vi "Flowmeter.vi"() -> ()   [LabVIEW 2017]
uses:
  Type Def/Data.ctl
  <vilib>/DAQmx/read.llb/DAQmx Read (Analog 2D DBL NChan NSamp).vi
  <vilib>/DAQmx/configure/timing.llb/DAQmx Timing (Sample Clock).vi
  <vilib>/DAQmx/miscellaneous.llb/DAQmx Fill In Error Info.vi
panel:
  out "valeur de l'horloge en ms":u32
  in  "Bouton Accueil":bool
  out "task out":refnum<k21>
  out "Type .EXE":bool
  out "sortie d'erreur 2":errorcluster caption="sortie d'erreur"
  out "error out":errorcluster
  out "Chaîne":string
  out "error IO":errorcluster
  out "sortie d'erreur":errorcluster
  in  "Start acquisition":bool
  out "High Voltage":dbl format="%#_2g"
  out "FLOW_SMC3":dbl caption="FLOW_AMP" format="%#.2g"
  out "FLOW_SMC2":dbl caption="FLOW_OSC" format="%#.2g"
  out "FLOW_SMC1":dbl caption="FLOW_BENCH" format="%#.2g"
  out "TEMP_SMC3":dbl caption="TEMP_AMP" format="%#.2g"
  out "TEMP_SMC2":dbl caption="TEMP_OSC" format="%#.2g"
  out "TEMP_SMC1":dbl caption="TEMP_BENCH" format="%#.2g"
  out "Flow data file (1sec)":refnum<file>
  out "Tableau":dbl[](array[numeric])
  in  "Stop":bool
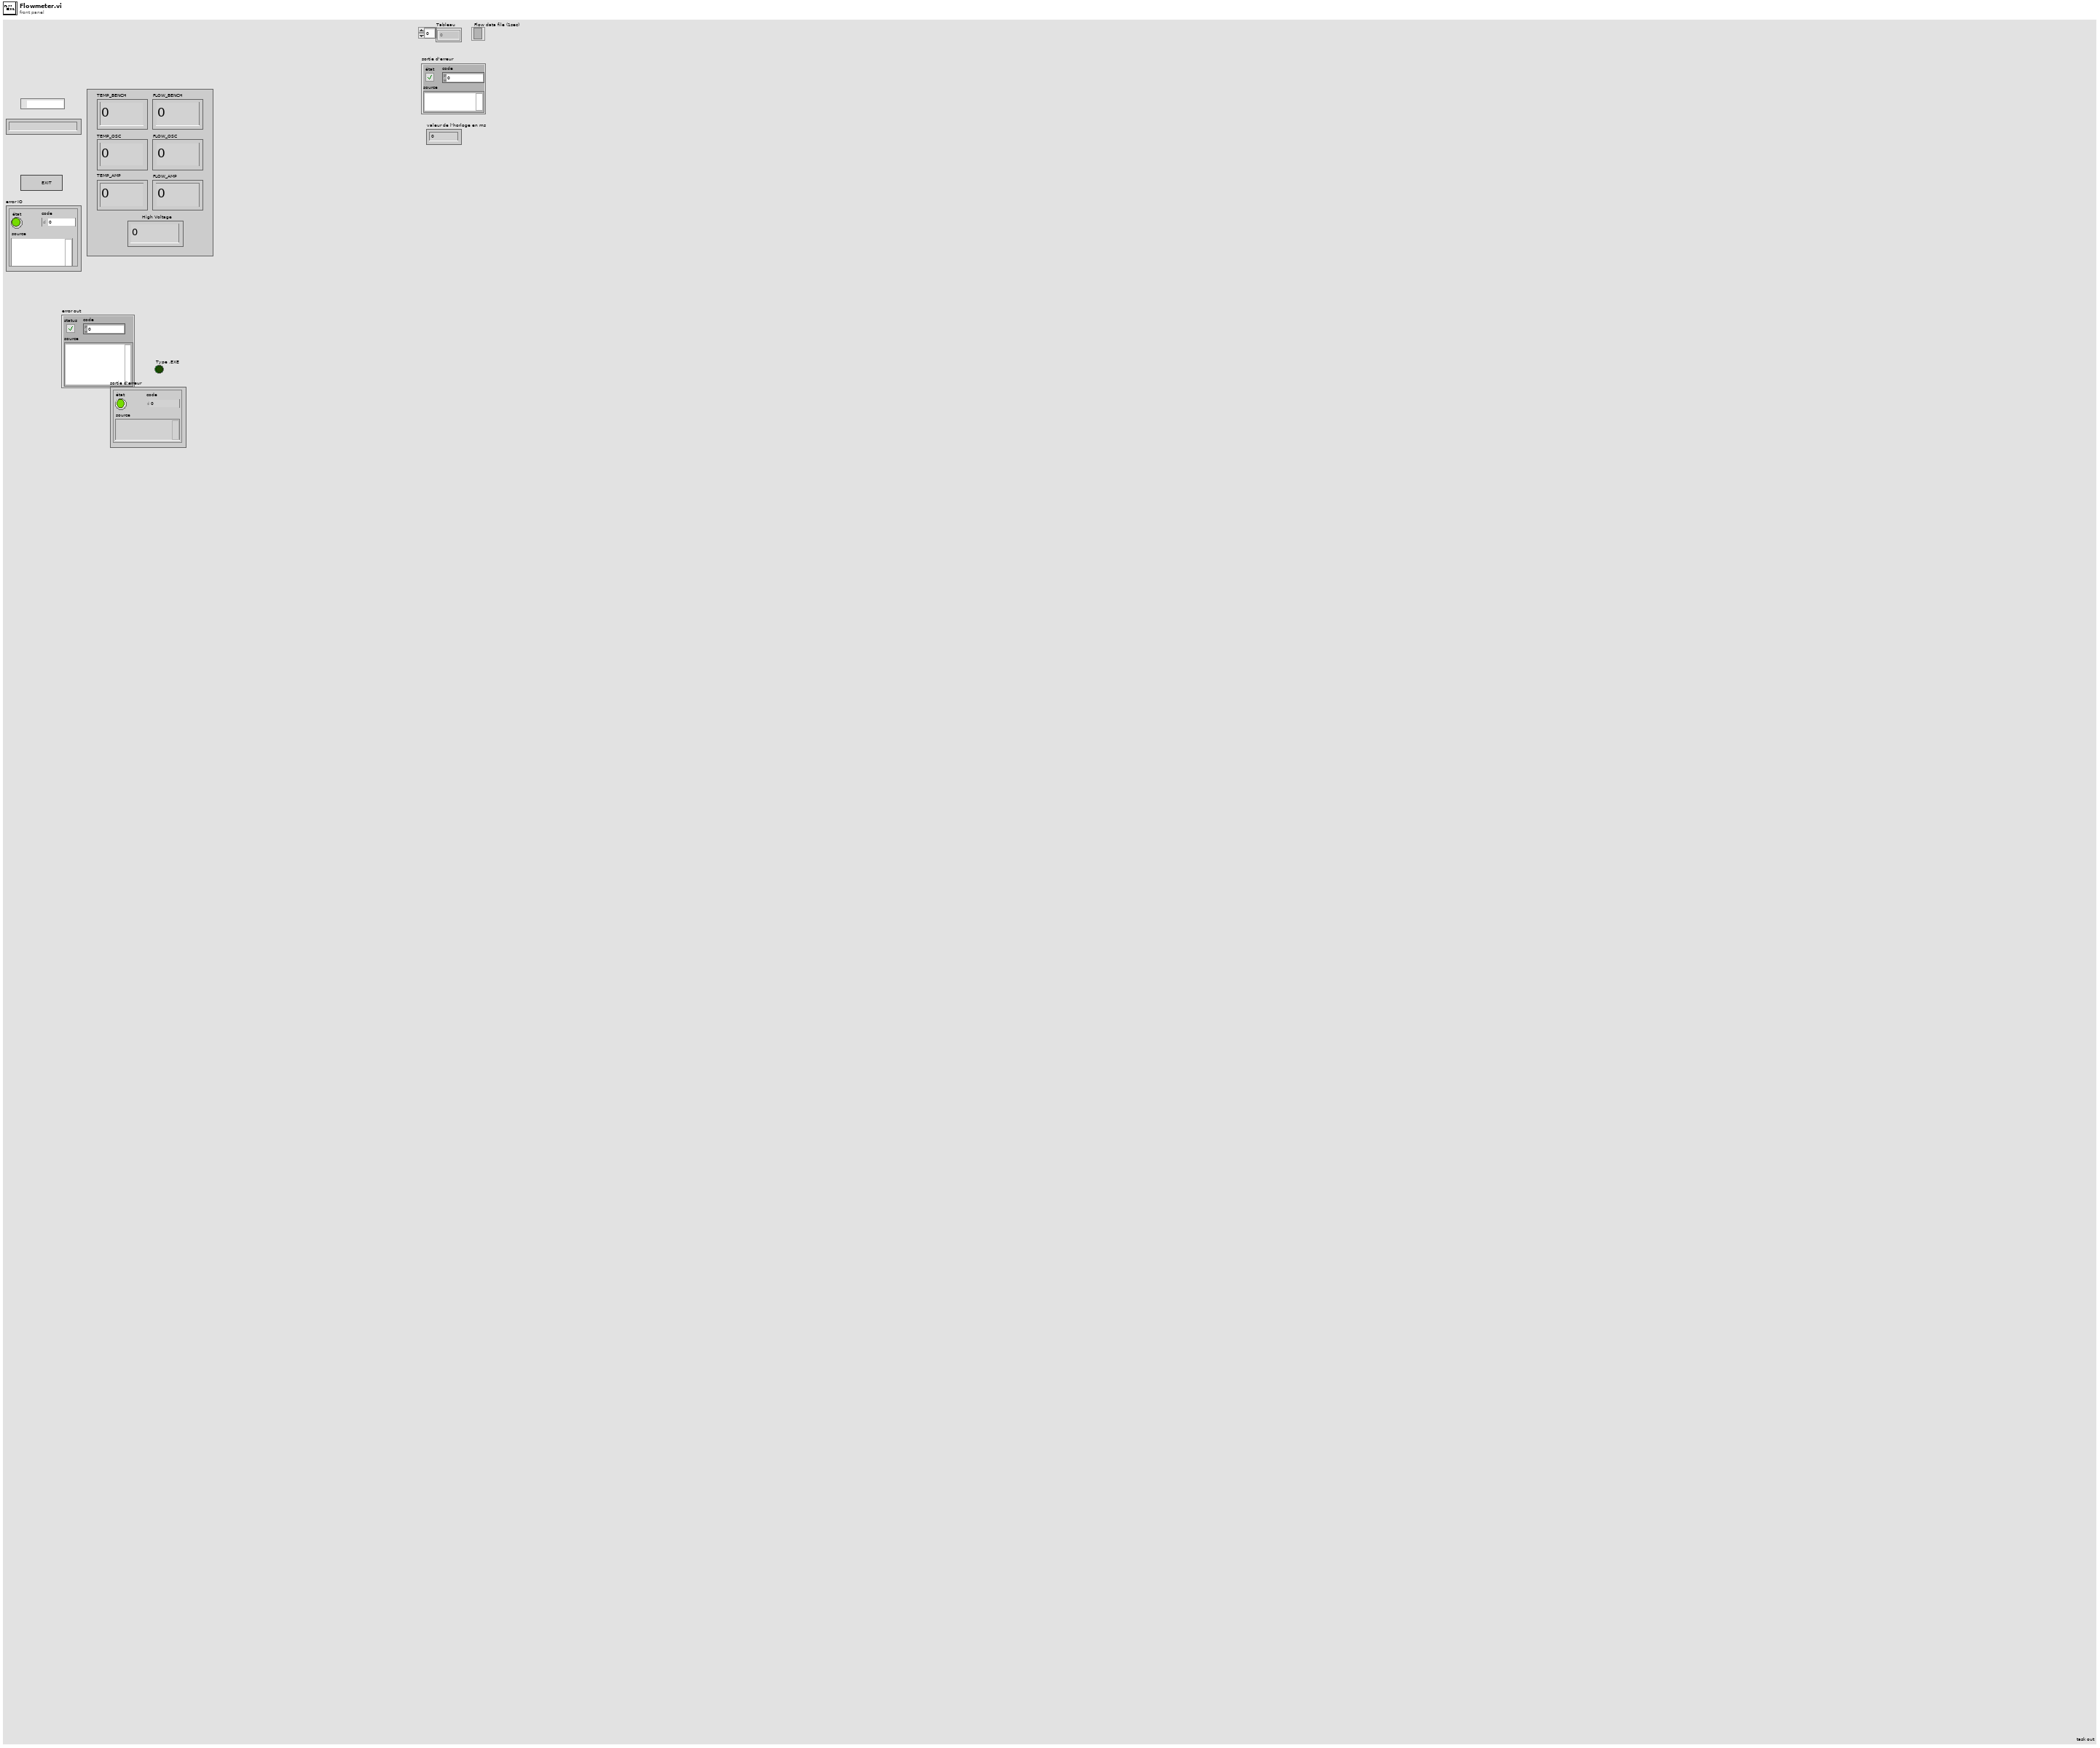
[diagram p1: front panel]
types:
  T1 = enum8{"Enabled", "Disabled", "Disabled and Grayed Out"}
  T2 = typedef "Data.ctl" = cluster{enum16{"Stop", "Read", "Init"}, dbl[][], "Date":string, "Time":dbl}
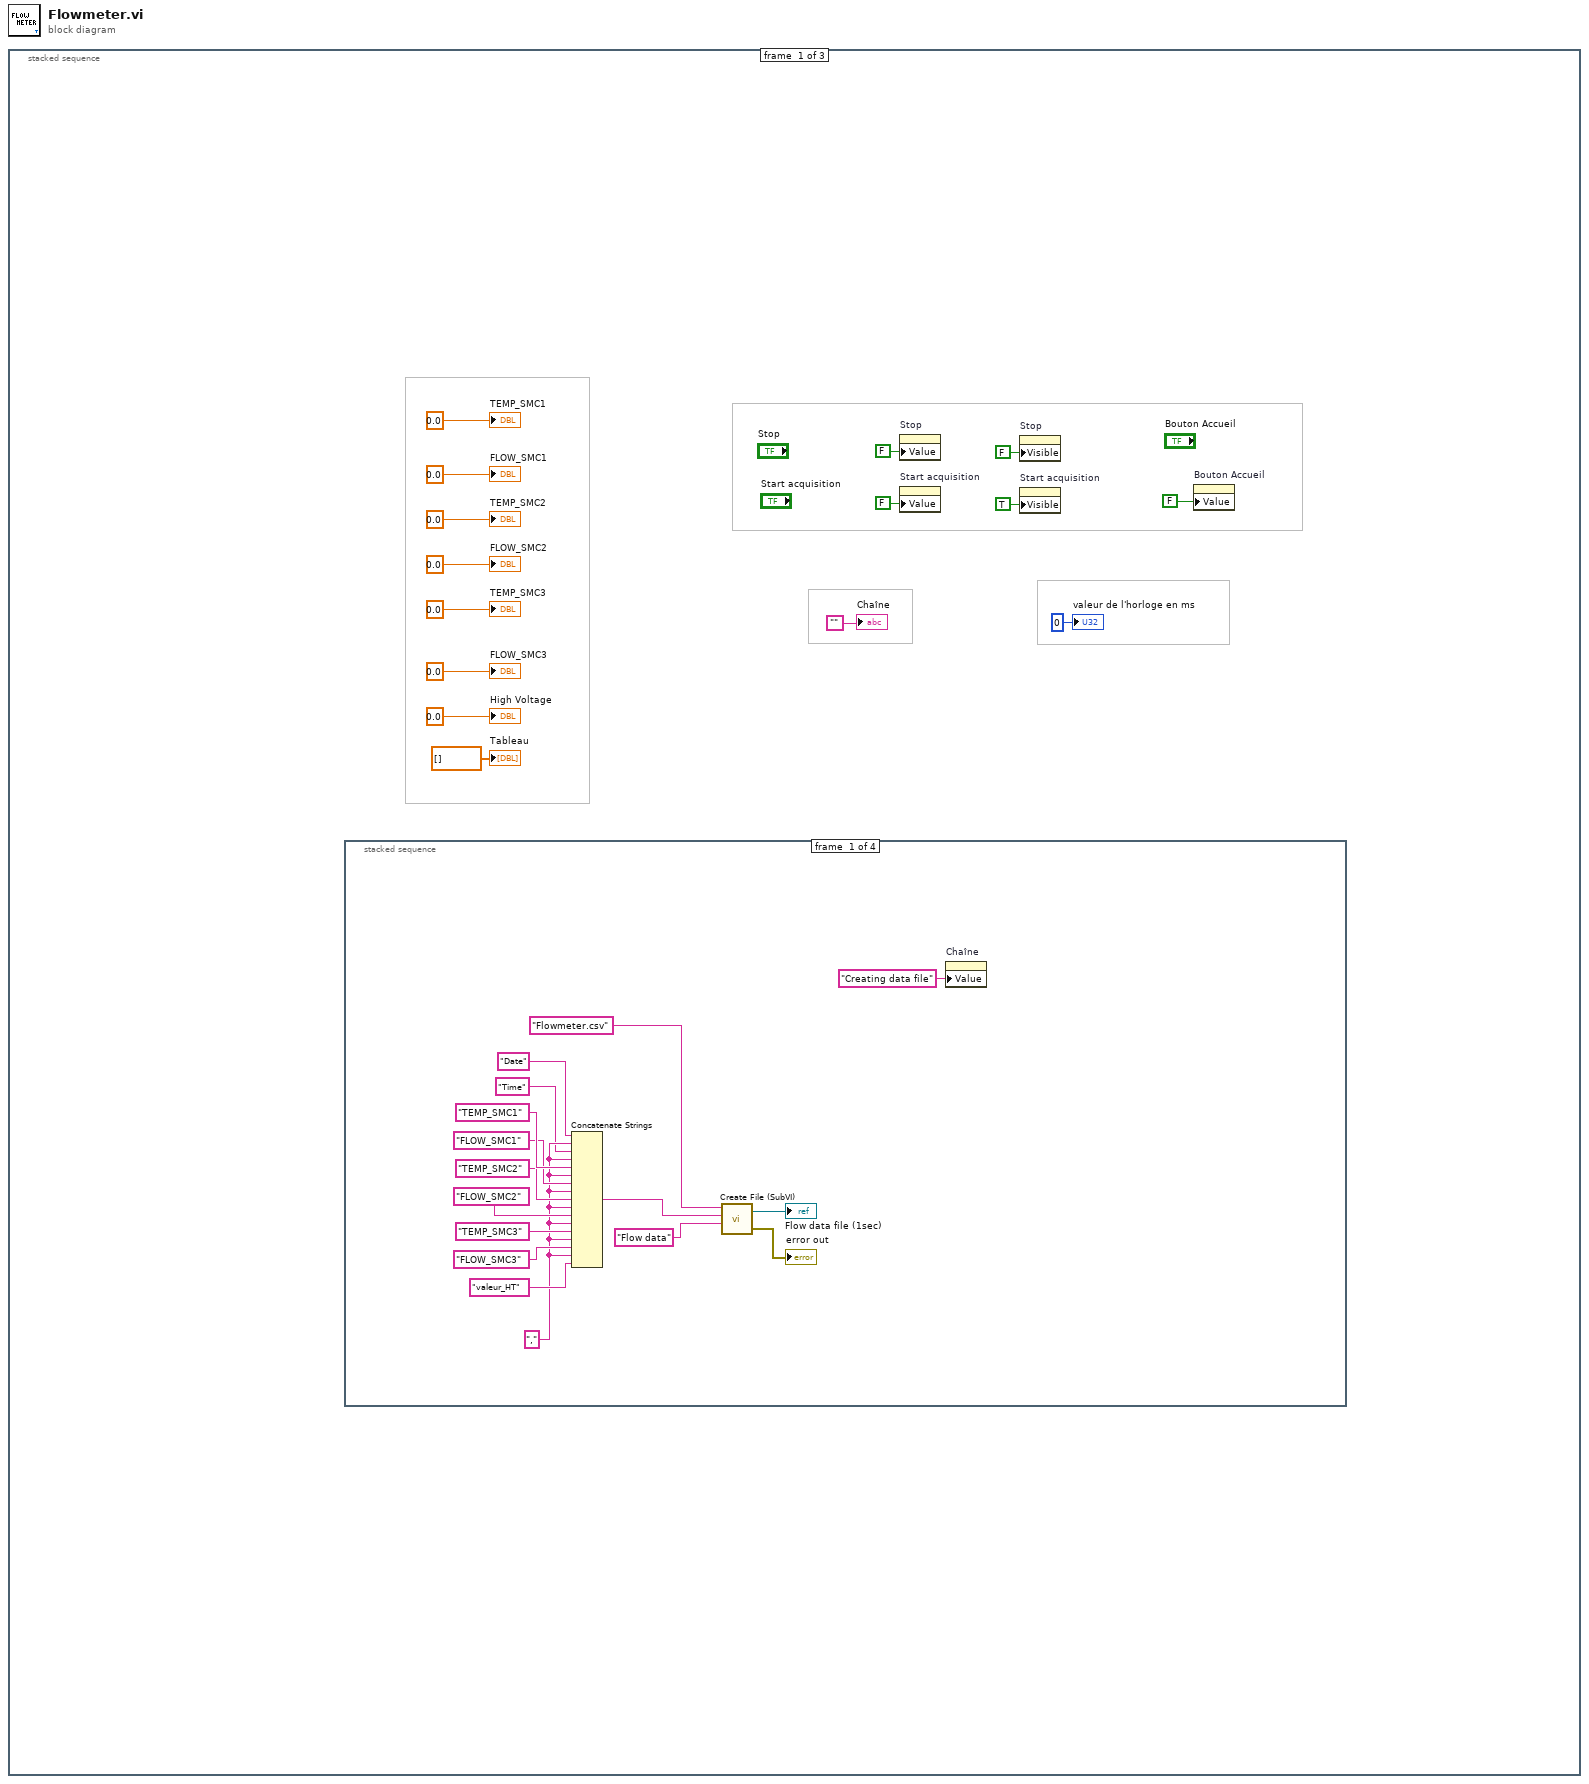
[diagram p0: block diagram]
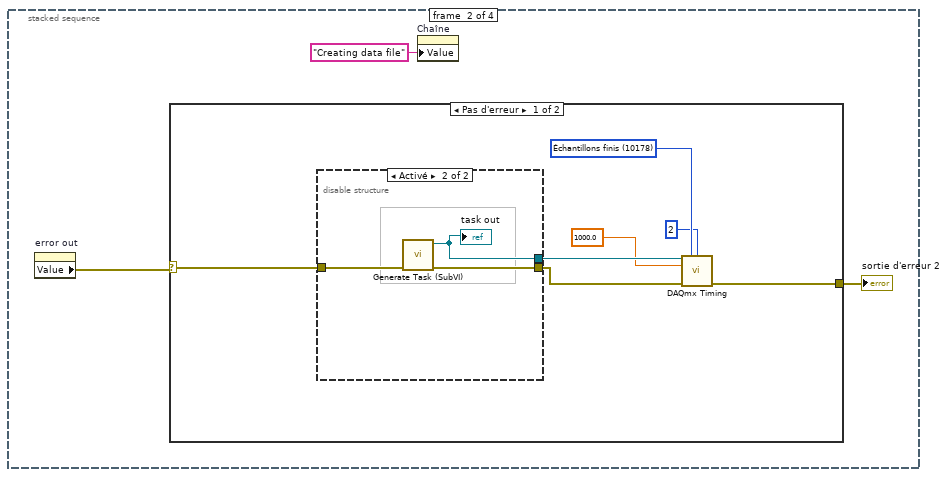
[diagram p2: hidden frame]
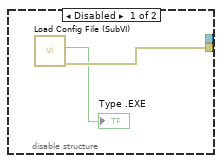
[diagram p3: hidden frame]
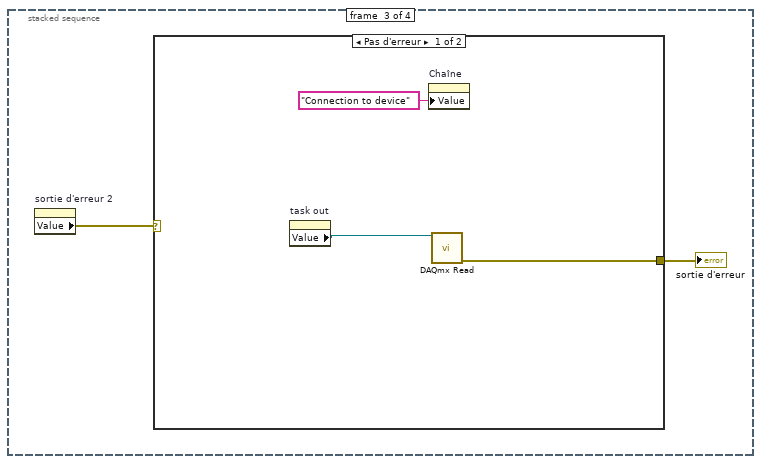
[diagram p5: hidden frame]
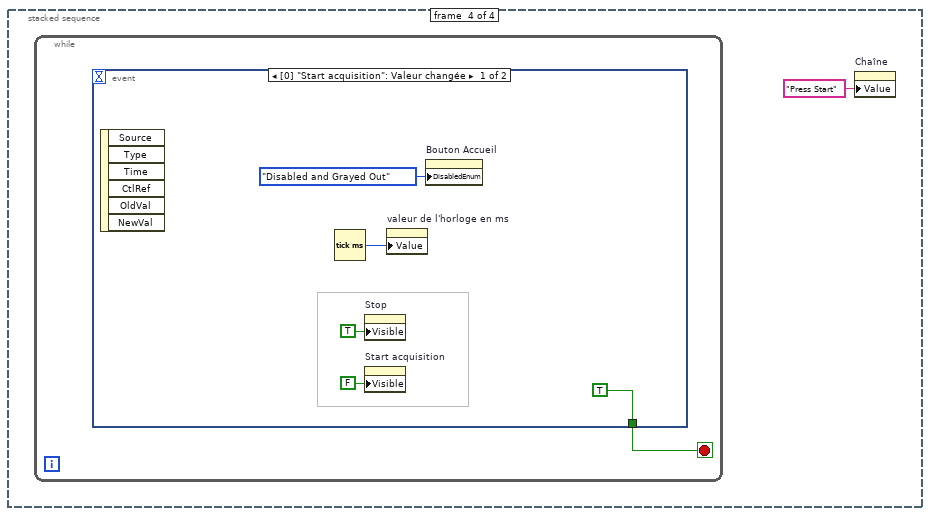
[diagram p7: hidden frame]
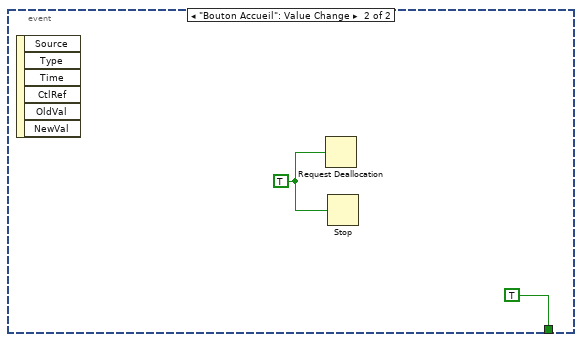
[diagram p8: hidden frame]
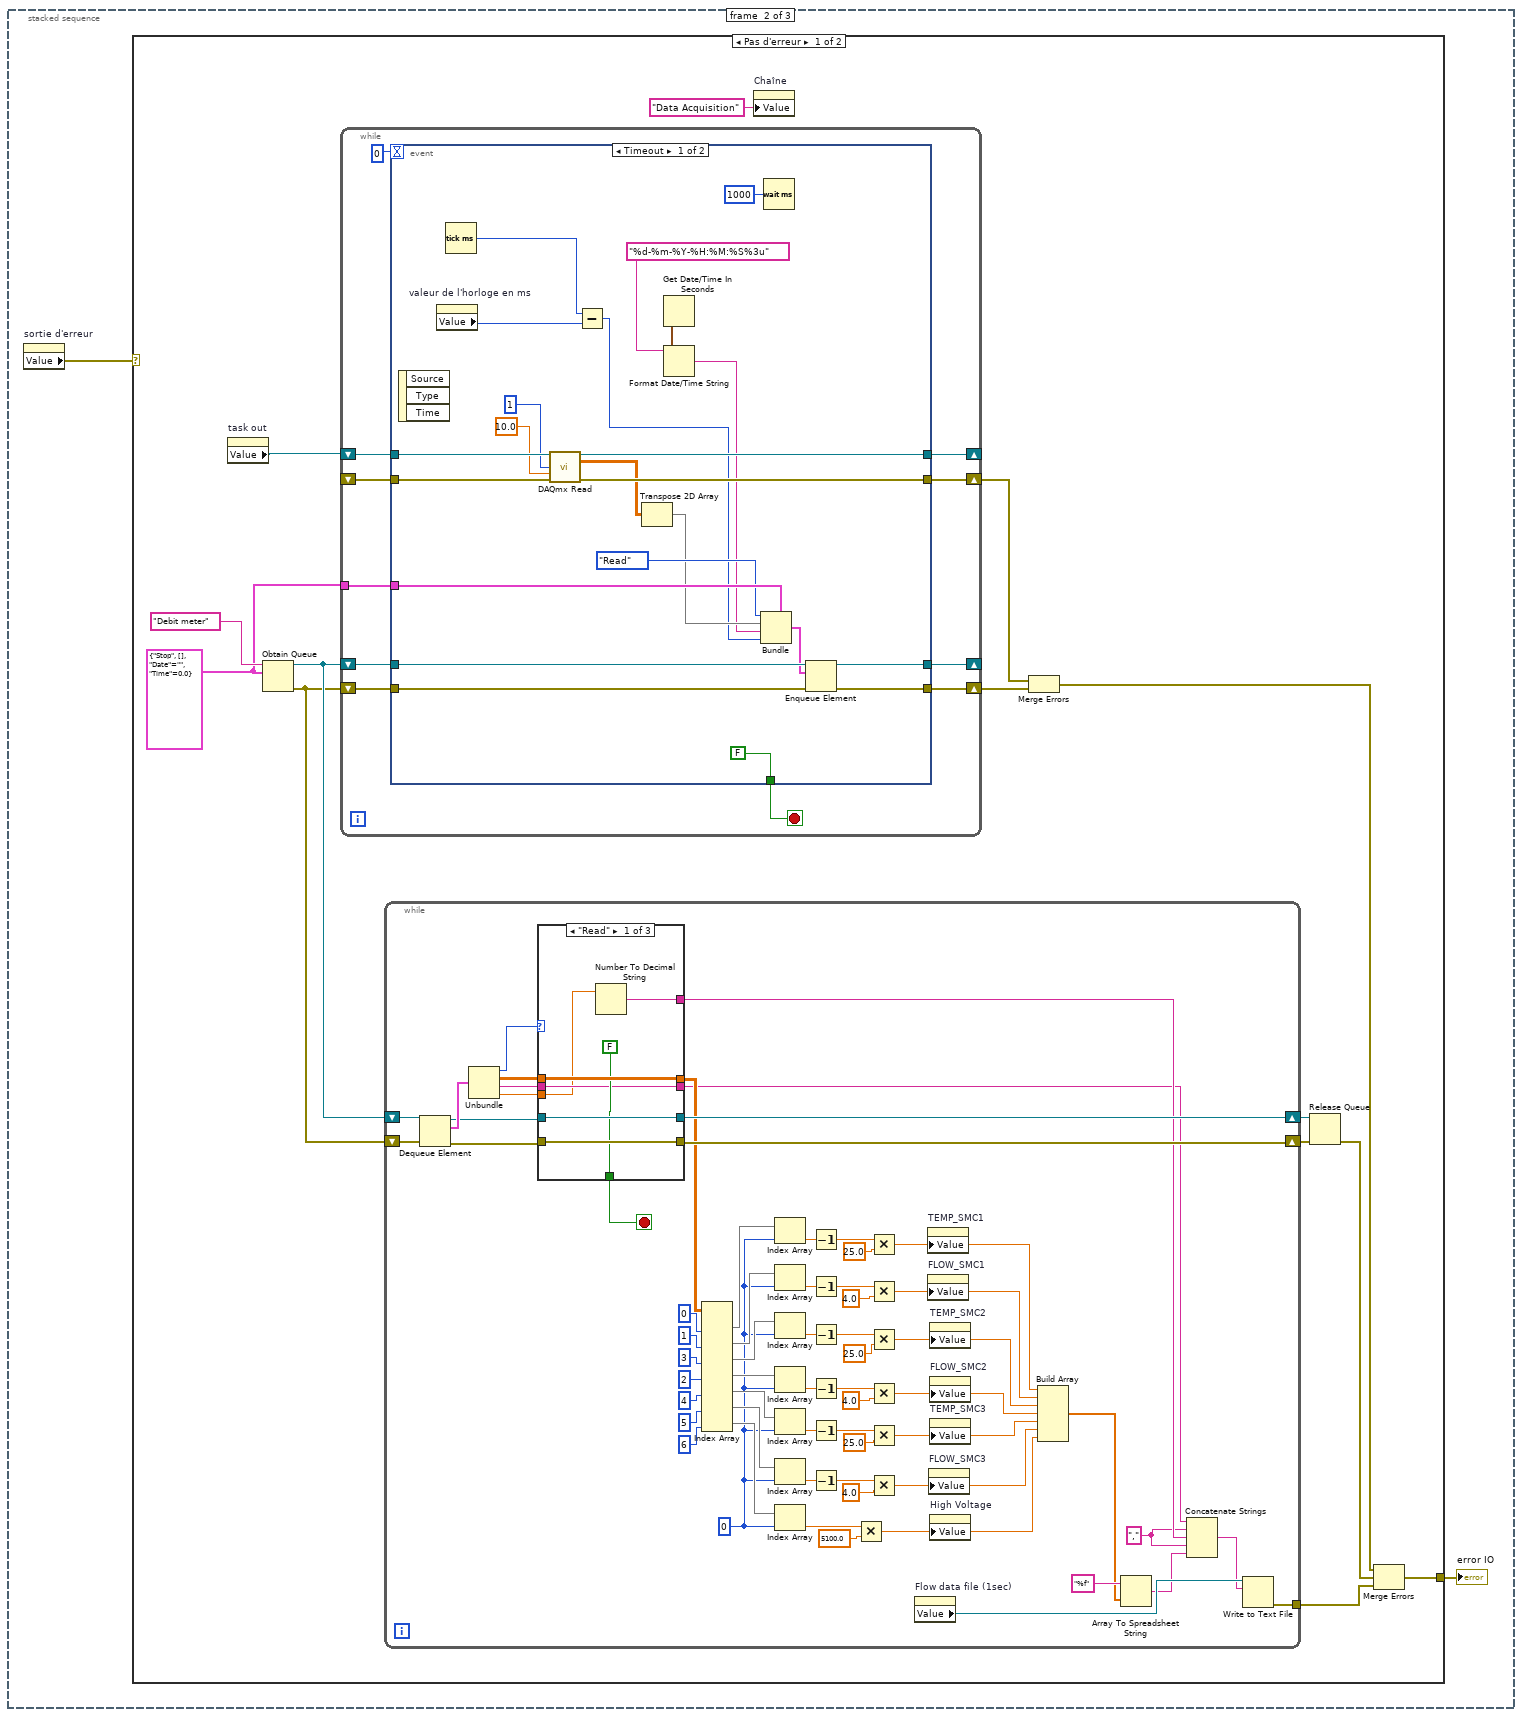
[diagram p9: hidden frame]
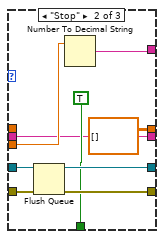
[diagram p10: hidden frame]
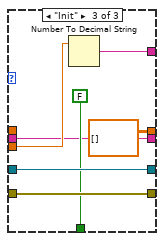
[diagram p11: hidden frame]
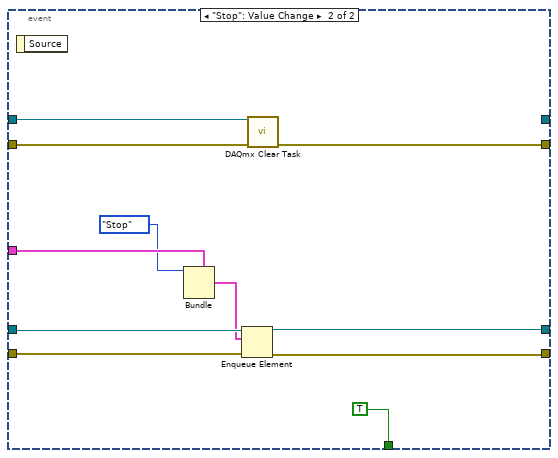
[diagram p12: hidden frame]
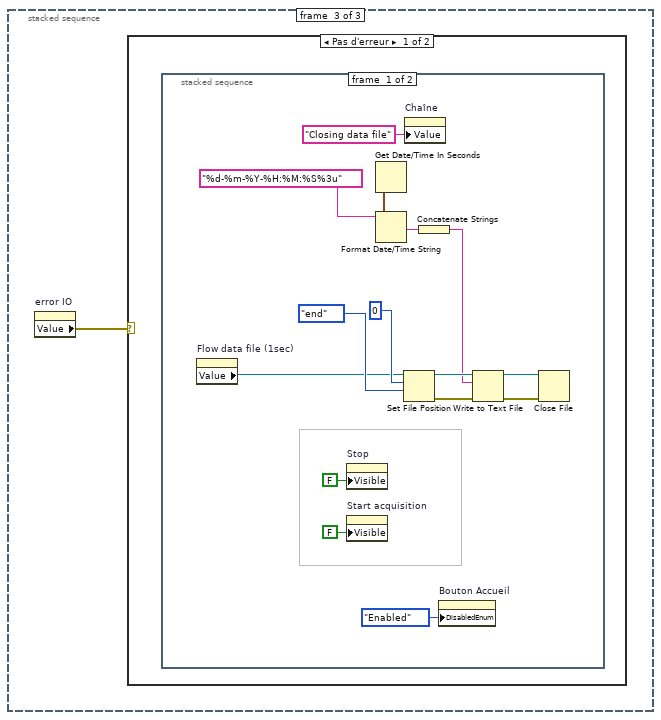
[diagram p14: hidden frame]
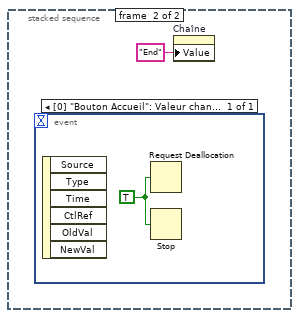
[diagram p15: hidden frame]
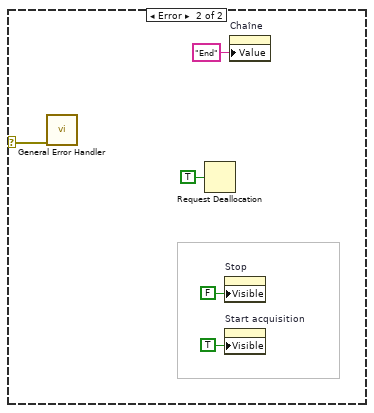
[diagram p16: hidden frame]
diagram:
  n1 = stacked-sequence {
    frame #0 {
      n2 = stacked-sequence {
        frame #0 {
          w18 = ","
          n3 = Concatenate Strings("Date" ("data name"), w18, "Time" ("data name"), w18, "TEMP_SMC1" ("data name"), w18, "FLOW_SMC1" ("data name"), w18, "TEMP_SMC2" ("data name"), w18, "FLOW_SMC2" ("data name"), w18, "TEMP_SMC3" ("data name"), w18, "FLOW_SMC3" ("data name"), w18, "valeur_HT" ("data name")) -> (w31:string)
          n4 = call "Create File (SubVI).vi"("headers"="Flow data", "data name"=w31, "file name"="Flowmeter.csv") -> ("error out"=→"error out":errorcluster, "Byte Stream File out"=→"Flow data file (1sec)":refnum<file>)  [unwired: 1 in]
          n5 = property on="Chaîne" class="Ch"("Value"="Creating data file" ("Chaîne")) -> ()  [unwired: 2 in, 2 out]
        }
        frame #1 {
          n6 = property on="error out" class="Clust (strict)"() -> ("Value"=w33:errorcluster)  [unwired: 2 in, 2 out]
          n7 = case shown="Pas d'erreur" w33 {
            selector: w33 -> [w40 w47]
            tunnel: [w41 w47] -> w32
            frame No Error {
              w37 = 10178 items=["Échantillons finis"=10178, "Échantillons continus"=10123, "Point par point avec cadencement matériel"=12522] ("sample mode")
              n8 = disable-structure shown="Activé" {
                disable-tunnel: [w43 w45] -> w39
                disable-tunnel: w40 -> [_ w46]
                disable-tunnel: [_ w44] -> w38
                frame Disabled {
                  n9 = call "Load Config File (SubVI).vi"() -> ("sortie d'erreur"=w43:errorcluster, "Type .EXE"=→"Type .EXE":bool)  [unwired: 9 in, 1 out]
                }
                frame Enabled {
                  n10 = call "Generate Task (SubVI).vi"("error in"=w46) -> ("error out"=w45:errorcluster, "task out"=w44:refnum<k21>)  [unwired: 9 in]
                  "task out" <- w44
                }
              }
              n11 = call-poly <vilib>:"DAQmx Timing.vi"("task/channels in"=w38, "sample mode"=w37, "samples per channel"=2, "rate"=1000.0, "error in"=w39) -> ("error out"=w41:errorcluster)  [unwired: 9 in, 1 out]
            }
            frame Error {
            }
          }
          "sortie d'erreur 2" <- w32
          n12 = property on="Chaîne" class="Ch"("Value"="Creating data file" ("Chaîne")) -> ()  [unwired: 2 in, 2 out]
        }
        frame #2 {
          n13 = property on="sortie d'erreur 2" class="Clust (strict)"() -> ("Value"=w49:errorcluster)  [unwired: 2 in, 2 out]
          n14 = case shown="Pas d'erreur" w49 {
            selector: w49 -> [_ w53]
            tunnel: [w50 w53] -> w48
            frame No Error {
              n15 = property on="task out" class="NomDAQmx (strict)"() -> ("Value"=w51:refnum<k21>)  [unwired: 2 in, 2 out]
              n16 = property on="Chaîne" class="Ch"("Value"="Connection to device" ("Chaîne")) -> ()  [unwired: 2 in, 2 out]
              n17 = call-poly <vilib>:"DAQmx Read.vi"("task/channels in"=w51) -> ("error out"=w50:errorcluster)  [unwired: 12 in, 2 out]
            }
            frame Error {
            }
          }
          "sortie d'erreur" <- w48
        }
        frame #3 {
          n18 = while {
            stop <- w55 stop-if-true
            n19 = event shown="[0] \"Start acquisition\": Valeur changée" {
              selector: _ -> [_ _]
              dyn-events: _ -> [_ _]
              timeout: _ -> [_ _]
              tunnel: [TRUE TRUE] -> w55
              event "Start acquisition": Value Change {
                n20 = event-data() -> ()  [unwired: 1 in, 6 out]
                n21 = Tick Count (ms)() -> (millisecond timer value=w56:u32)
                n22 = property on="Stop" class="Bool (strict)"("Visible"=TRUE ("Bouton Stop")) -> ()  [unwired: 2 in, 2 out]
                n23 = property on="Start acquisition" class="Bool (strict)"("Visible"=FALSE ("Start acquisition")) -> ()  [unwired: 2 in, 2 out]
                n24 = property on="valeur de l'horloge en ms" class="NumNb (strict)"("Value"=w56) -> ()  [unwired: 2 in, 2 out]
                n25 = property on="Bouton Accueil" class="Bool (strict)"("DisabledEnum"=T1."Disabled and Grayed Out" ("Désactivé")) -> ()  [unwired: 2 in, 2 out]
              }
              event "Bouton Accueil": Value Change {
                w61 = TRUE
                n26 = event-data() -> ()  [unwired: 1 in, 6 out]
                n27 = Request Deallocation(w61) -> ()
                n28 = Stop(stop? (T)=w61) -> ()
              }
            }
          }
          n29 = property on="Chaîne" class="Ch"("Value"="Press Start" ("Chaîne")) -> ()  [unwired: 2 in, 2 out]
        }
      }
      n30 = property on="Stop" class="Bool (strict)"("Value"=FALSE ("Bouton Stop")) -> ()  [unwired: 2 in, 2 out]
      n31 = property on="Start acquisition" class="Bool (strict)"("Value"=FALSE ("Start acquisition")) -> ()  [unwired: 2 in, 2 out]
      n32 = property on="Stop" class="Bool (strict)"("Visible"=FALSE ("Bouton Stop")) -> ()  [unwired: 2 in, 2 out]
      n33 = property on="Start acquisition" class="Bool (strict)"("Visible"=TRUE ("Start acquisition")) -> ()  [unwired: 2 in, 2 out]
      n34 = property on="Bouton Accueil" class="Bool (strict)"("Value"=FALSE ("Bouton Accueil")) -> ()  [unwired: 2 in, 2 out]
      "TEMP_SMC1" <- 0.0 ("TEMP_SMC1")
      "TEMP_SMC2" <- 0.0 ("TEMP_SMC2")
      "TEMP_SMC3" <- 0.0 ("TEMP_SMC3")
      "FLOW_SMC1" <- 0.0 ("FLOW_SMC1")
      "FLOW_SMC2" <- 0.0 ("FLOW_SMC2")
      "FLOW_SMC3" <- 0.0 ("FLOW_SMC3")
      "High Voltage" <- 0.0 ("valeur HT")
      "Tableau" <- dbl[] [] ("Tableau")
      "Chaîne" <- ""
      "valeur de l'horloge en ms" <- u32 0 ("valeur de l'horloge en ms")
    }
    frame #1 {
      n35 = property on="sortie d'erreur" class="Clust (strict)"() -> ("Value"=w64:errorcluster)  [unwired: 2 in, 2 out]
      n36 = case shown="Pas d'erreur" w64 {
        selector: w64 -> [_ w211]
        tunnel: [w67 w211] -> w63
        frame No Error {
          w73 = T2 {enum."Stop", [], "Date"="", "Time"=0.0}
          n37 = property on="task out" class="NomDAQmx (strict)"() -> ("Value"=w65:refnum<k21>)  [unwired: 2 in, 2 out]
          n38 = Obtain Queue(name (unnamed)="Debit meter" ("nom (aucun)"), element data type=w73) -> (queue out=w77:refnum<queue>, error out=w76:errorcluster)  [unwired: 3 in, 1 out]
          n39 = while {
            shift-right: [w173] -> _
            shift-left: w77 -> [w175]
            shift-right: [w174] -> w71
            shift-left: w76 -> [w176]
            tunnel: w73 -> [w171]
            shift-right: [w166] -> _
            shift-left: w65 -> [w170]
            shift-right: [w167] -> w70
            shift-left: _ -> [w169]
            stop <- w172 stop-if-true
            n40 = event shown="[0] Timeout" {
              selector: _ -> [_ _]
              dyn-events: _ -> [_ _]
              timeout: 0 -> [_ _]
              tunnel: w176 -> [w198 w210]
              tunnel: w175 -> [w199 w207]
              tunnel: [w197 w209] -> w174
              tunnel: [w196 w208] -> w173
              tunnel: [FALSE TRUE] -> w172
              tunnel: w171 -> [w193 w205]
              tunnel: w170 -> [w192 w201]
              tunnel: w169 -> [w191 w202]
              tunnel: [w188 w200] -> w167
              tunnel: [w184 _] -> w166
              event Timeout {
                n41 = event-data() -> ()  [unwired: 1 in, 3 out]
                n42 = property on="valeur de l'horloge en ms" class="NumNb (strict)"() -> ("Value"=w181:u32)  [unwired: 2 in, 2 out]
                n43 = Tick Count (ms)() -> (millisecond timer value=w180:u32)
                n44 = call-poly <vilib>:"DAQmx Read.vi"("task/channels in"=w192, "number of samples per channel"=1, "timeout"=10.0, "error in"=w191) -> ("task out"=w184:refnum<k21>, "data"=w186:dbl[][], "error out"=w188:errorcluster)  [unwired: 9 in]
                n45 = Subtract(x=w180, y=w181) -> (x-y=w178:u32)
                n46 = Transpose 2D Array(2D array=w186) -> (transposed array=w185:dbl[][])
                n47 = Get Date/Time In Seconds() -> (seconds since 1Jan1904=w183:timestamp)
                n48 = Format Date/Time String(time format string (%c)="%d-%m-%Y-%H:%M:%S%3u", seconds (now)=w183) -> (date/time string=w179:string)  [unwired: 1 in]
                n49 = Bundle(cluster=w193, enum16{"Stop", "Read", "Init"}."Read", w185, "Date"=w179, "Time"=w178) -> (w194:T2)
                n50 = Wait (ms)(milliseconds to wait=u32 1000 ("attente (ms)")) -> ()  [unwired: 1 out]
                n51 = Enqueue Element(queue=w199, element=w194, error in (no error)=w198) -> (queue out=w196:refnum<queue>, error out=w197:errorcluster)  [unwired: 1 in, 1 out]
              }
              event "Stop": Value Change {
                n52 = event-data() -> ()  [unwired: 1 in, 1 out]
                n53 = Bundle(cluster=w205, enum16{"Stop", "Read", "Init"}."Stop") -> (w206:T2)  [unwired: 3 in]
                n54 = Enqueue Element(queue=w207, element=w206, error in (no error)=w210) -> (queue out=w208:refnum<queue>, error out=w209:errorcluster)  [unwired: 1 in, 1 out]
                n55 = call <vilib>:"DAQmx Clear Task.vi"("task in"=w201, "error in"=w202) -> ("error out"=w200:errorcluster)  [unwired: 13 in]
              }
            }
          }
          n56 = while {
            shift-right: [w134] -> w74
            shift-left: w77 -> [w141]
            shift-right: [w135] -> w75
            shift-left: w76 -> [w142]
            tunnel: [w87] -> w68
            stop <- w113 stop-if-true
            w82 = ","
            w97 = 0 ("indice désactivé (col)")
            n57 = Dequeue Element(queue=w141, error in (no error)=w142) -> (queue out=w137:refnum<queue>, element=w140:T2, error out=w136:errorcluster)  [unwired: 1 in, 1 out]
            n58 = Unbundle(w140) -> (w139:enum16{"Stop", "Read", "Init"}, w138:dbl[][], "Date"=w80:string, "Time"=w79:dbl)
            n59 = case shown="\"Read\"" w139 {
              tunnel: w138 -> [w147 _ _]
              tunnel: w137 -> [w149 w158 w165]
              tunnel: w136 -> [w148 w157 w164]
              tunnel: [w148 w156 w164] -> w135
              tunnel: [w149 w155 w165] -> w134
              tunnel: [w147 dbl[][] [] dbl[][] []] -> w112
              tunnel: [FALSE TRUE FALSE] -> w113
              tunnel: [w145 w152 w161] -> w83
              tunnel: [w144 w150 w159] -> w81
              tunnel: w80 -> [w144 w150 w159]
              tunnel: w79 -> [w143 w151 w160]
              frame "Read" {
                n60 = Number To Decimal String(number=w143) -> (decimal integer string=w145:string)  [unwired: 1 in]
              }
              frame "Stop" {
                n61 = Flush Queue(queue=w158, error in (no error)=w157) -> (queue out=w155:refnum<queue>, error out=w156:errorcluster)  [unwired: 1 out]
                n62 = Number To Decimal String(number=w151) -> (decimal integer string=w152:string)  [unwired: 1 in]
              }
              frame "Init" {
                n63 = Number To Decimal String(number=w160) -> (decimal integer string=w161:string)  [unwired: 1 in]
              }
            }
            n64 = Index Array(array=w112, index (col) #1=0 ("indice désactivé (col)"), index (col) #2=1 ("indice (col)"), index (col) #3=3 ("indice (col)"), index (col) #4=2 ("indice (col)"), index (col) #5=4 ("indice (col)"), index (col) #6=5 ("indice (col)"), index (col) #7=6 ("indice (col)")) -> (element #1=w122:dbl[], element #2=w128:dbl[], element #3=w125:dbl[], element #4=w130:dbl[], element #5=w126:dbl[], element #6=w132:dbl[], element #7=w133:dbl[])  [unwired: 7 in]
            n65 = Index Array(array=w122, index=w97) -> (element=w104:dbl)
            n66 = Index Array(array=w128, index=w97) -> (element=w103:dbl)
            n67 = Index Array(array=w125, index=w97) -> (element=w102:dbl)
            n68 = Index Array(array=w130, index=w97) -> (element=w101:dbl)
            n69 = Index Array(array=w126, index=w97) -> (element=w100:dbl)
            n70 = Index Array(array=w132, index=w97) -> (element=w99:dbl)
            n71 = Index Array(array=w133, index=w97) -> (element=w98:dbl)
            n72 = Decrement(x=w104) -> (x-1=w121:dbl)
            n73 = Decrement(x=w103) -> (x-1=w127:dbl)
            n74 = Decrement(x=w102) -> (x-1=w123:dbl)
            n75 = Decrement(x=w101) -> (x-1=w129:dbl)
            n76 = Decrement(x=w100) -> (x-1=w124:dbl)
            n77 = Decrement(x=w99) -> (x-1=w131:dbl)
            n78 = Multiply(x=w98, y=5100.0) -> (x*y=w90:dbl)
            n79 = Multiply(x=w121, y=25.0) -> (x*y=w96:dbl)
            n80 = Multiply(x=w127, y=4.0) -> (x*y=w95:dbl)
            n81 = Multiply(x=w123, y=25.0) -> (x*y=w94:dbl)
            n82 = Multiply(x=w129, y=4.0) -> (x*y=w93:dbl)
            n83 = Multiply(x=w124, y=25.0) -> (x*y=w92:dbl)
            n84 = Multiply(x=w131, y=4.0) -> (x*y=w91:dbl)
            n85 = property on="Flow data file (1sec)" class="Ref (strict)"() -> ("Value"=w88:refnum<file>)  [unwired: 2 in, 2 out]
            n86 = property on="TEMP_SMC1" class="NumNb (strict)"("Value"=w96) -> ()  [unwired: 2 in, 2 out]
            n87 = property on="FLOW_SMC1" class="NumNb (strict)"("Value"=w95) -> ()  [unwired: 2 in, 2 out]
            n88 = property on="FLOW_SMC3" class="NumNb (strict)"("Value"=w91) -> ()  [unwired: 2 in, 2 out]
            n89 = property on="TEMP_SMC2" class="NumNb (strict)"("Value"=w94) -> ()  [unwired: 2 in, 2 out]
            n90 = property on="FLOW_SMC2" class="NumNb (strict)"("Value"=w93) -> ()  [unwired: 2 in, 2 out]
            n91 = property on="TEMP_SMC3" class="NumNb (strict)"("Value"=w92) -> ()  [unwired: 2 in, 2 out]
            n92 = property on="High Voltage" class="NumNb (strict)"("Value"=w90) -> ()  [unwired: 2 in, 2 out]
            n93 = Build Array(w96, w95, w94, w93, w92, w91, w90) -> (w86:dbl[])
            n94 = Array To Spreadsheet String(array=w86, 3:"%f" ("chaîne de format")) -> (spreadsheet string=w85:string)  [unwired: 1 in]
            n95 = Concatenate Strings(w81, w82, w83, w82, w85) -> (w84:string)
            n96 = Write to Text File(file (use dialog)=w88, text=w84) -> (error out=w87:errorcluster)  [unwired: 2 in, 2 out]
          }
          n97 = property on="Chaîne" class="Ch"("Value"="Data Acquisition" ("Chaîne")) -> ()  [unwired: 2 in, 2 out]
          n98 = Merge Errors(w70, w71) -> (w69:errorcluster)
          n99 = Release Queue(queue=w74, error in (no error)=w75) -> (error out=w72:errorcluster)  [unwired: 1 in, 2 out]
          n100 = Merge Errors(w69, w72, w68) -> (w67:errorcluster)
        }
        frame Error {
        }
      }
      "error IO" <- w63
    }
    frame #2 {
      n101 = property on="error IO" class="Clust (strict)"() -> ("Value"=w212:errorcluster)  [unwired: 2 in, 2 out]
      n102 = case shown="Pas d'erreur" w212 {
        selector: w212 -> [_ w232]
        frame No Error {
          n103 = stacked-sequence {
            frame #0 {
              n104 = property on="Flow data file (1sec)" class="Ref (strict)"() -> ("Value"=w219:refnum<file>)  [unwired: 2 in, 2 out]
              n105 = property on="Stop" class="Bool (strict)"("Visible"=FALSE ("Bouton Stop")) -> ()  [unwired: 2 in, 2 out]
              n106 = property on="Start acquisition" class="Bool (strict)"("Visible"=FALSE ("Start acquisition")) -> ()  [unwired: 2 in, 2 out]
              n107 = Get Date/Time In Seconds() -> (seconds since 1Jan1904=w225:timestamp)
              n108 = Format Date/Time String(time format string (%c)="%d-%m-%Y-%H:%M:%S%3u", seconds (now)=w225) -> (date/time string=w223:string)  [unwired: 1 in]
              n109 = Set File Position(offset (in bytes) (0)=i64 0 ("offset (en octets) (0)"), refnum=w219, from (0:start)=enum16{"start", "end", "current"}."end" ("à partir de (0 : start)")) -> (refnum out=w226:refnum<file>, error out=w215:errorcluster)  [unwired: 1 in]
              n110 = property on="Chaîne" class="Ch"("Value"="Closing data file" ("Chaîne")) -> ()  [unwired: 2 in, 2 out]
              n111 = Concatenate Strings(w223) -> (w222:string)
              n112 = property on="Bouton Accueil" class="Bool (strict)"("DisabledEnum"=T1."Enabled" ("Désactivé")) -> ()  [unwired: 2 in, 2 out]
              n113 = Write to Text File(file (use dialog)=w226, text=w222, error in=w215) -> (refnum out=w227:refnum<file>, error out=w214:errorcluster)  [unwired: 1 in, 1 out]
              n114 = Close File(refnum=w227, error in=w214) -> ()  [unwired: 2 out]
            }
            frame #1 {
              n115 = event shown="[0] \"Bouton Accueil\": Valeur changée" {
                selector: _ -> [_]
                dyn-events: _ -> [_]
                timeout: _ -> [_]
                event "Bouton Accueil": Value Change {
                  w229 = TRUE ("flag")
                  n116 = event-data() -> ()  [unwired: 1 in, 6 out]
                  n117 = Request Deallocation(w229) -> ()
                  n118 = Stop(stop? (T)=w229) -> ()
                }
              }
              n119 = property on="Chaîne" class="Ch"("Value"="End" ("Chaîne")) -> ()  [unwired: 2 in, 2 out]
            }
          }
        }
        frame Error {
          n120 = call <vilib>:"General Error Handler.vi"("error in (no error)"=w232) -> ()  [unwired: 10 in, 5 out]
          n121 = Request Deallocation(TRUE ("flag")) -> ()
          n122 = property on="Stop" class="Bool (strict)"("Visible"=FALSE ("Bouton Stop")) -> ()  [unwired: 2 in, 2 out]
          n123 = property on="Start acquisition" class="Bool (strict)"("Visible"=TRUE ("Start acquisition")) -> ()  [unwired: 2 in, 2 out]
          n124 = property on="Chaîne" class="Ch"("Value"="End" ("Chaîne")) -> ()  [unwired: 2 in, 2 out]
        }
      }
    }
  }
